vi "Check and Override Channel Configuration.vi"(8 "error in (no error)":errorcluster, 10 "Custom Config Data in":u8[](array[numeric]) format="%.0x", 11 "CIFFIFO in":refnum<class "CIF_CIPC_Fifo_U8.lvclass">) -> (0 "error out":errorcluster, 2 "Custom Config Data out":u8[](array[numeric]) format="%.0x", 3 "CIFFIFO out":refnum<class "CIF_CIPC_Fifo_U8.lvclass">)   [LabVIEW 2021, in "CIF_CIPC_Fifo_U8.lvclass"]
uses:
  CIF_CIPC_Fifo_U8.lvclass
  CIF_CIPC_Fifo_U8.lvclass/CIF_CIPC_Fifo_U8.ctl
  ChannelCommon/ChannelCommon.lvlib
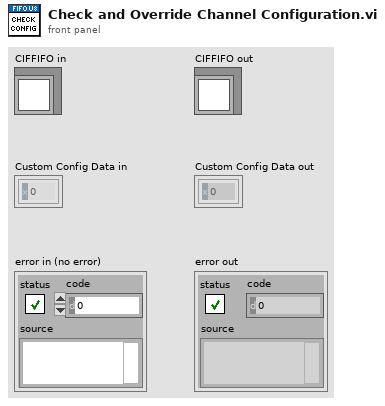
[diagram p1: front panel]
types:
  T1 = typedef "ChannelCommon.lvlib/FIFO Config.ctl" = cluster{"Max Bytes/Msg":u64, "Max Msg/FIFO":u64, "Flags":u64, "Custom Data":u8[]}
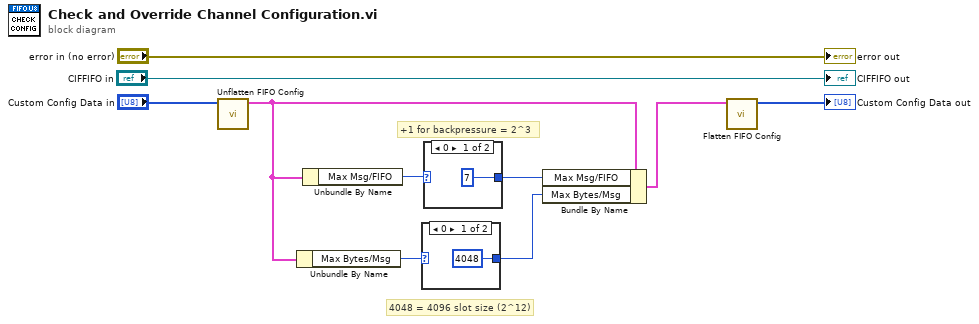
[diagram p0: block diagram]
diagram:
  # "+1 for backpressure = 2^3"
  # "4048 = 4096 slot size (2^12)"
  n1 = call "Unflatten FIFO Config.vi"("Flattened Data in"="Custom Config Data in") -> ("FIFO Config out"=w5:T1)  [unwired: 9 in, 1 out]
  n2 = Unbundle By Name(w5) -> ("Max Bytes/Msg"=w7:u64)
  n3 = Unbundle By Name(w5) -> ("Max Msg/FIFO"=w6:u64)
  n4 = case shown="0" w7 {
    selector: w7 -> [_ w12]
    tunnel: [u64 4048 ("y") w12] -> w2
    frame 0 {
    }
    frame 1, Default {
    }
  }
  n5 = case shown="0" w6 {
    selector: w6 -> [_ w14]
    tunnel: [u64 7 ("y") w14] -> w3
    frame 0 {
    }
    frame 1, Default {
    }
  }
  n6 = Bundle By Name(cluster=w5, "Max Msg/FIFO"=w3, "Max Bytes/Msg"=w2) -> (w4:T1)
  n7 = call "Flatten FIFO Config.vi"("FIFO Config in"=w4) -> ("Flattened FIFO Config"=→"Custom Config Data out":u8[])  [unwired: 10 in]
  "error out" <- "error in (no error)"
  "CIFFIFO out" <- "CIFFIFO in"
